vi "GetRectAndLineIntersectionFloat.vi"(4 "Y2 In":sgl, 6 "X2 In":sgl, 8 "No Error":errorcluster, 9 "Y1 In":sgl, 10 "X1 In":sgl, 11 "Rect":T1) -> (0 "Error Out":errorcluster, 1 "Y1 Out":sgl, 2 "X1 Out":sgl, 3 "Intersect?":bool, 5 "Y2 Out":sgl, 7 "X2 Out":sgl)   [LabVIEW 2024, in "SDL3.lvlib" / "Rect.lvlib"]
doc: "<B>Summary</B>\nCalculate the intersection of a rectangle and line segment with float precision.\n\n<B>Remarks</B>\nThis function is used to clip a line segment to a rectangle. A line segment contained entirely within the rectangle or that does not intersect will remain unchanged. A line segment that crosses the rectangle at either or both ends will be clipped to the boundary of the rectangle and the new coordinates saved in X1, Y1, X2, and/or Y2 as necessary."
uses:
  Rect.lvlib
  FRect--cluster.ctl
  Lib/SDL3-32.dll
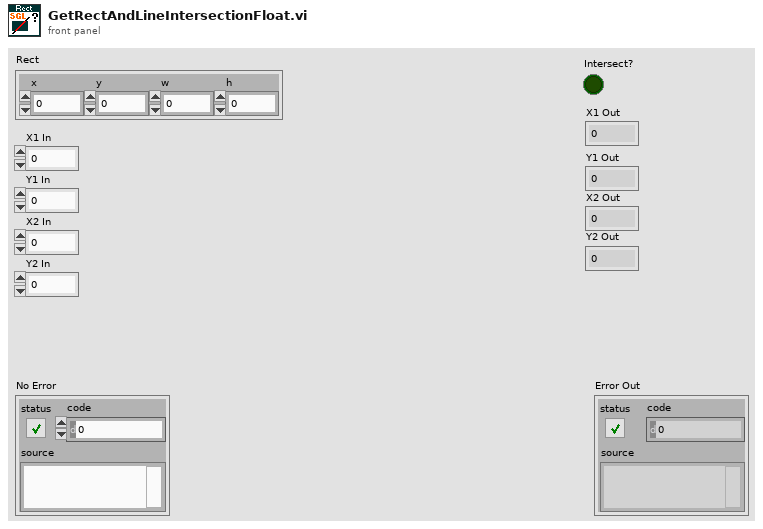
[diagram p1: front panel]
types:
  T1 = typedef "SDL3.lvlib/Rect.lvlib/FRect--cluster.ctl" = cluster{"x":sgl, "y":sgl, "w":sgl, "h":sgl}
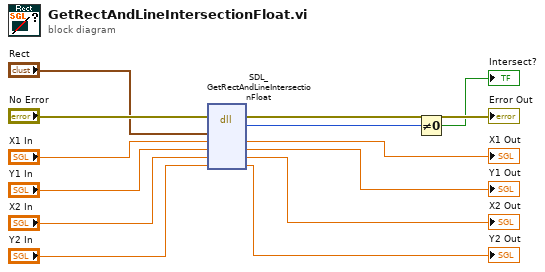
[diagram p0: block diagram]
diagram:
  n1 = dll-call lib="C:/Users/Thomas/Documents/Projects/LV-SDL3/Lib/SDL3-*.*" fn="SDL_GetRectAndLineIntersectionFloat"(error in="No Error", "rect"="Rect", "X1"="X1 In", "Y1"="Y1 In", "X2"="X2 In", "Y2"="Y2 In") -> (error out=→"Error Out":errorcluster, "return type"=w11:i32, "X1"=→"X1 Out":sgl, "Y1"=→"Y1 Out":sgl, "X2"=→"X2 Out":sgl, "Y2"=→"Y2 Out":sgl)  [unwired: 3 in, 1 out]
  n2 = Not Equal To 0?(x=w11) -> (x != 0?=→"Intersect?":bool)
